vi "Test Remove Invalid Characters.vi"() -> ()   [LabVIEW 2025]
uses:
  Controls/Character Position Possible Letters.ctl
  <vilib>/addons/_JKI Toolkits/Caraya/classes/Assert/Assert Equal Value_Variant.vi
  <vilib>/addons/_JKI Toolkits/Caraya/classes/Test/Test.lvclass
  <vilib>/addons/_JKI Toolkits/Caraya/classes/Assert/Assert.lvclass
  Libraries/WordleSolver/WordleSolver.lvlib
panel:
  out "Updated Character Position":string[](array[string])
  out "error out":errorcluster
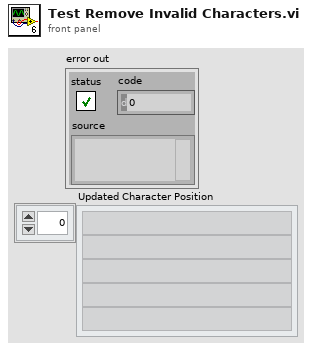
[diagram p1: front panel]
types:
  T1 = typedef "Character Position Possible Letters.ctl" = string[]
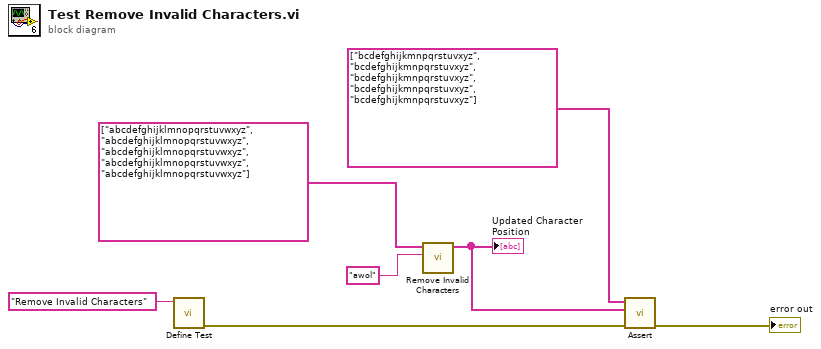
[diagram p0: block diagram]
diagram:
  n1 = call <vilib>:"Define Test.vi"("Label (VI Title)"="Remove Invalid Characters") -> ("error out"=w7:errorcluster)  [unwired: 9 in, 1 out]
  n2 = call "Remove Invalid Characters.vi"("String"="awol", "Character Position Possible Letters"=T1 ["abcdefghijklmnopqrstuvwxyz", "abcdefghijklmnopqrstuvwxyz", "abcdefghijklmnopqrstuvwxyz", "abcdefghijklmnopqrstuvwxyz", "abcdefghijklmnopqrstuvwxyz"]) -> ("Updated Character Position"=w1:string[])  [unwired: 9 in]
  "Updated Character Position" <- w1
  n3 = call-poly <vilib>:"Assert.vi"("error in (no error)"=w7, "Actual"=w1, "Expected"=T1 ["bcdefghijkmnpqrstuvxyz", "bcdefghijkmnpqrstuvxyz", "bcdefghijkmnpqrstuvxyz", "bcdefghijkmnpqrstuvxyz", "bcdefghijkmnpqrstuvxyz"] ("Character Position Possible Letters")) -> ("error out"=→"error out":errorcluster)  [unwired: 7 in, 1 out]
